vi "Map Control References.vi"(8 "error in (no error)":errorcluster, 11 "Engine in":refnum<class "Engine.lvclass">) -> (0 "error out":errorcluster, 3 "Engine out":refnum<class "Engine.lvclass">)   [LabVIEW 2023, in "Engine.lvlib" / "Engine.lvclass"]
doc: "<b>Map Control References </b>\nThis routine calls <b> Collect Control References </b> then <b>Link Control References</b>\n\nThe purpose of this routine is to pack control references into the calling class and reduce the amount of coding necessary to collect references in private data.\n\nThis routine is called by default in the <b>Post Launch Initialize</b> routine"
uses:
  Library/Engine.lvclass
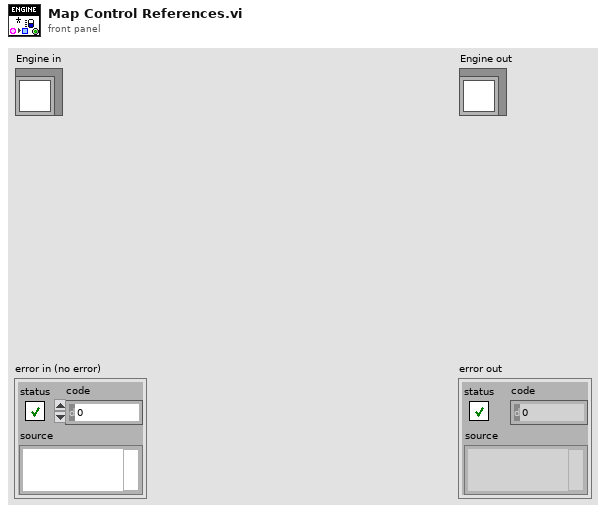
[diagram p1: front panel]
types:
  T1 = cluster{"Ctl Refnum":refnum<vi>, "Label.Text":string}[]
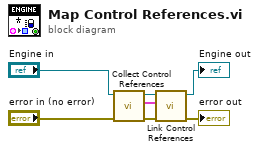
[diagram p0: block diagram]
diagram:
  n1 = call "Collect Control References.vi"("error in (no error)"="error in (no error)", "Engine in"="Engine in") -> ("error out"=w6:errorcluster, "Control References"=w5:T1, "Engine out"=w4:refnum<class "Engine.lvclass">)  [unwired: 7 in]
  n2 = call-dynamic "Link Control References.vi"("error in (no error)"=w6, "Control References"=w5, "Engine in"=w4) -> ("error out"=→"error out":errorcluster, "Engine out"=→"Engine out":refnum<class "Engine.lvclass">)  [unwired: 7 in]
